vi "Build Cleanup Scripting.vi"(8 "error in (no error)":errorcluster, 9 "Dynamic":bool, 10 "VI Refnum":refnum<vi>, 11 "Scaffold Project Refs In":T1) -> (0 "error out":errorcluster)   [LabVIEW 2018, in "LVClassByRef.lvlib"]
uses:
  <resource>/Framework/Providers/LVClassByRef/LVClassByRef.lvlib
  <resource>/Framework/Providers/LVClassByRef/Scaffold Project Refs.ctl
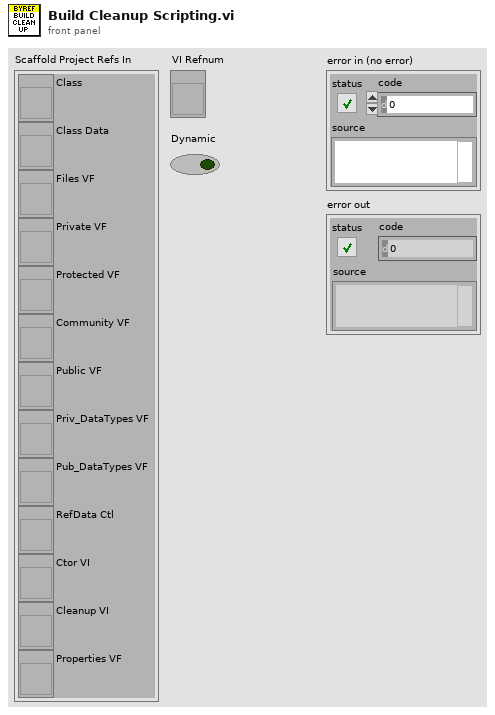
[diagram p1: front panel]
types:
  T1 = typedef "LVClassByRef.lvlib/Scaffold Project Refs.ctl" = cluster{"Class":refnum<vi>, "Class Data":refnum<vi>, "Files VF":refnum<vi>, "Private VF":refnum<vi>, "Protected VF":refnum<vi>, "Community VF":refnum<vi>, "Public VF":refnum<vi>, "Priv_DataTypes VF":refnum<vi>, "Pub_DataTypes VF":refnum<vi>, "RefData Ctl":refnum<vi>, "Ctor VI":refnum<vi>, "Cleanup VI":refnum<vi>, "Properties VF":refnum<vi>}
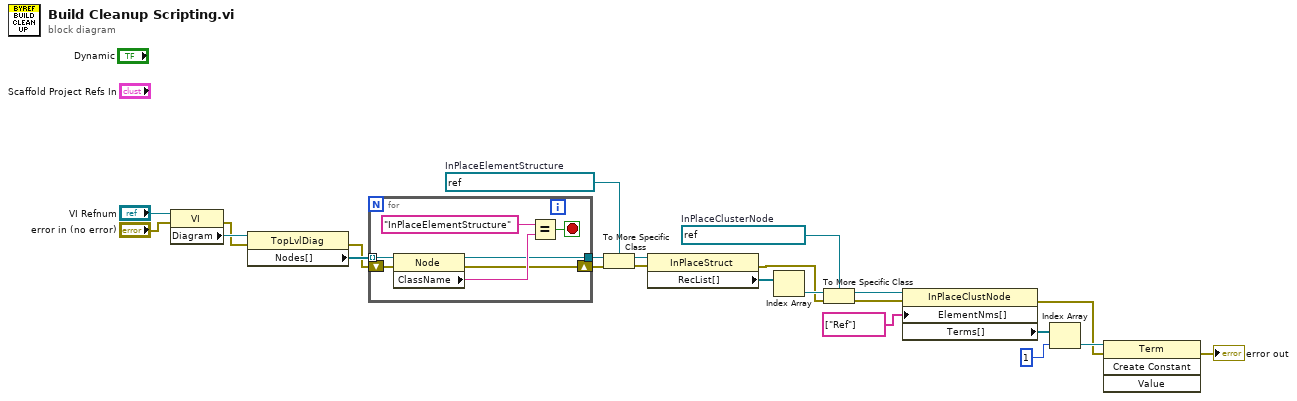
[diagram p0: block diagram]
diagram:
  w4 = refnum<vi> refnum  # InPlaceClusterNode
  w20 = refnum<vi> refnum  # InPlaceElementStructure
  n1 = property on="Property Node" class="VI"(reference="VI Refnum", error in="error in (no error)") -> (error out=w16:errorcluster, "Diagram"=w23:refnum<vi>)  [unwired: 1 out]
  n2 = property on="Property Node" class="TopLvlDiag"(reference=w23, error in=w16) -> (error out=w14:errorcluster, "Nodes[]"=w22:refnum<vi>[])  [unwired: 1 out]
  n3 = for {
    tunnel: w22 -> [w30] mode=indexing
    tunnel: [w26] -> w21
    shift-right: [w24] -> w13
    shift-left: w14 -> [w25]
    stop <- w27 stop-if-true
    n4 = property class="Node"(reference=w30, error in=w25) -> (reference out=w26:refnum<vi>, error out=w24:errorcluster, "ClassName"=w28:string)
    n5 = Equal?(x="InPlaceElementStructure", y=w28) -> (x = y?=w27:bool)
  }
  n6 = To More Specific Class(target class=w20, reference=w21, error in=w13) -> (specific class reference=w19:refnum<vi>, error out=w12:errorcluster)
  n7 = property class="InPlaceStruct"(reference=w19, error in=w12) -> (error out=w5:errorcluster, "RecList[]"=w15:refnum<vi>[])  [unwired: 1 out]
  n8 = Index Array(array=w15) -> (element=w6:refnum<vi>)  [unwired: 1 in]
  n9 = To More Specific Class(target class=w4, reference=w6, error in=w5) -> (specific class reference=w3:refnum<vi>, error out=w2:errorcluster)
  n10 = property class="InPlaceClustNode"(reference=w3, error in=w2, "ElementNms[]"=string[] ["Ref"] ("Element Names[]")) -> (error out=w8:errorcluster, "Terms[]"=w11:refnum<vi>[])  [unwired: 1 out]
  n11 = Index Array(array=w11, index=1) -> (element=w9:refnum<vi>)
  n12 = invoke class="Term" method="Create Constant"(reference=w9, error in=w8) -> (error out=→"error out":errorcluster)  [unwired: 2 in, 3 out]
